vi "Read sensor ID.vi"(8 "error in (no error)":errorcluster, 11 "channel config object in":refnum<class "channel config object.lvclass">) -> (0 "error out":errorcluster, 2 "sensor ID":string, 3 "channel config object out":refnum<class "channel config object.lvclass">)   [LabVIEW 2013, in "channel config object.lvclass"]
uses:
  channel config object.lvclass
  channel config object.lvclass/channel config object.ctl
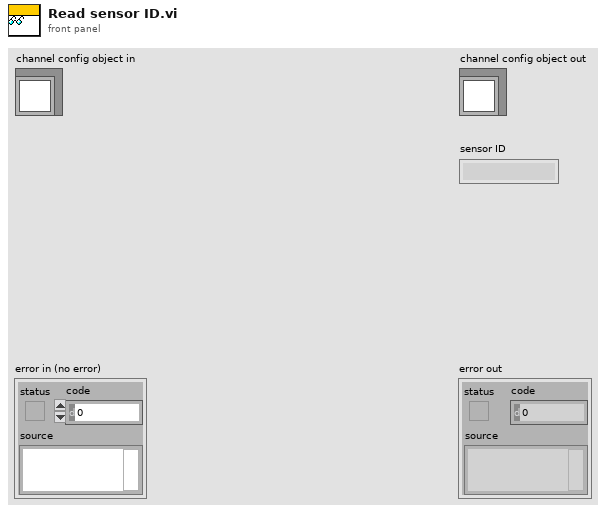
[diagram p1: front panel]
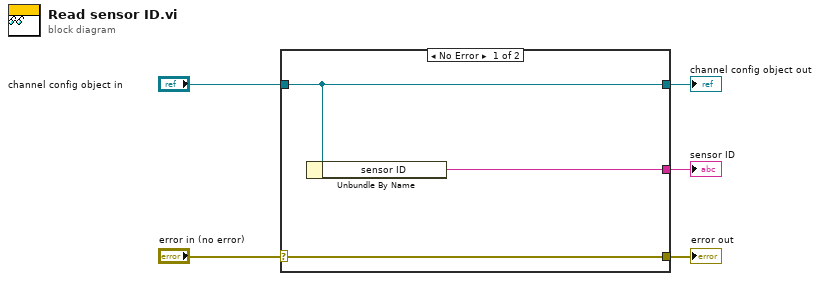
[diagram p0: block diagram]
diagram:
  n1 = case shown="No Error" "error in (no error)" {
    selector: "error in (no error)" -> [w8 w9]
    tunnel: [w8 w9] -> w4
    tunnel: [w7 w10] -> w2
    tunnel: "channel config object in" -> [w7 w10]
    tunnel: [w6 _] -> w1
    frame No Error {
      n2 = Unbundle By Name(w7) -> ("sensor ID"=w6:string)
    }
    frame Error {
    }
  }
  "error out" <- w4
  "channel config object out" <- w2
  "sensor ID" <- w1
